vi "Initialize.vi"(8 "error in (no error)":errorcluster, 11 "PID Loop in":refnum<class "PID Loop.lvclass">) -> (0 "error out":errorcluster, 3 "PID Loop out":refnum<class "PID Loop.lvclass">)   [LabVIEW 2024, in "PID Loop.lvlib" / "PID Loop.lvclass"]
uses:
  PID Loop.lvclass
  PID Loop.lvclass/PID Loop.ctl
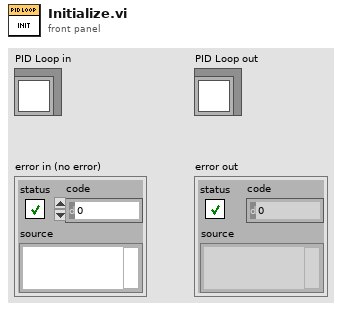
[diagram p1: front panel]
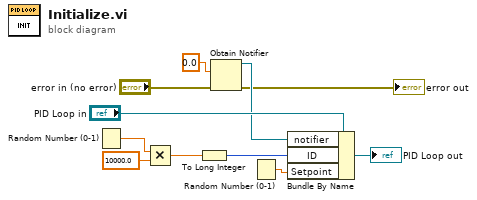
[diagram p0: block diagram]
diagram:
  n1 = Random Number (0-1)() -> (number: 0 to 1=w5:dbl)
  n2 = Multiply(x=w5, y=10000.0) -> (x*y=w3:dbl)
  n3 = To Long Integer(number=w3) -> (32bit integer=w2:i32)
  n4 = Obtain Notifier(notification data type=0.0, error in (no error)="error in (no error)") -> (notifier out=w9:refnum<notifier>, error out=→"error out":errorcluster)  [unwired: 2 in, 1 out]
  n5 = Random Number (0-1)() -> (number: 0 to 1=w1:dbl)
  n6 = Bundle By Name(cluster="PID Loop in", "notifier"=w9, "ID"=w2, "Setpoint"=w1) -> (→"PID Loop out":refnum<class "PID Loop.lvclass">)
